vi "Autonomous Independent.vi"() -> ()   [LabVIEW 2018]
doc: "This VI is called when autonomous begins, and will automatically be terminated when autonomous ends. You can carry out timed or sensor driven robot movement independently without needing to return to the caller."
uses:
  <vilib>/Rock Robotics/WPI/RobotDrive/WPI_RobotDriveArcadeDrive_Standard(NoSaturation).vi
  <vilib>/Rock Robotics/Network Tables/NT Write Numeric Array.vi
  Robot Global Data.vi
  <vilib>/Rock Robotics/Network Tables/NT Read String.vi
panel:
  in  "Encoders":T1
  in  "PID Gains":T2={"X PID"={"proportional gain (Kc)"=0.02000000000000001, "integral time (Ti, min)"=0.0, "derivative time (Td, min)"=0.0}, "Y PID"={"proportional gain (Kc)"=0.02000000000000001, "integral time (Ti, min)"=0.0, "derivative time (Td, min)"=0.0}, "Z PID"={"proportional gain (Kc)"=0.02000000000000001, "integral time (Ti, min)"=0.0, "derivative time (Td, min)"=0.0}} {"Z PID"."derivative time (Td, min)" format="%.3f"; "Z PID"."integral time (Ti, min)" format="%.3f"; "Z PID"."proportional gain (Kc)" format="%.3f"; "Y PID"."derivative time (Td, min)" format="%.3f"; "Y PID"."integral time (Ti, min)" format="%.3f"; "Y PID"."proportional gain (Kc)" format="%.3f"; "X PID"."derivative time (Td, min)" format="%.3f"; "X PID"."integral time (Ti, min)" format="%.3f"; "X PID"."proportional gain (Kc)" format="%.3f"}
  out "Current Movement, for debugging":T3 {"Y Joystick Value" scale=1.0..-1.0; "X Joystick Value" scale=-1.0..1.0}
  in  "Array of robot movements":T4(array[cluster])=[{"X Joystick Value"=0.39393939393939403, "Y Joystick Value"=0.0, "Delay (sec)"=1.0, "Movement Name"="turn"}, {"X Joystick Value"=-0.3737373737373737, "Y Joystick Value"=0.0, "Delay (sec)"=1.0, "Movement Name"="turn back"}] {"Y Joystick Value" scale=1.0..-1.0; "X Joystick Value" scale=-1.0..1.0}
  # "Be sure to right-click and choose Data Operations>>Make Current Value default if you want to save the array values with the VI"
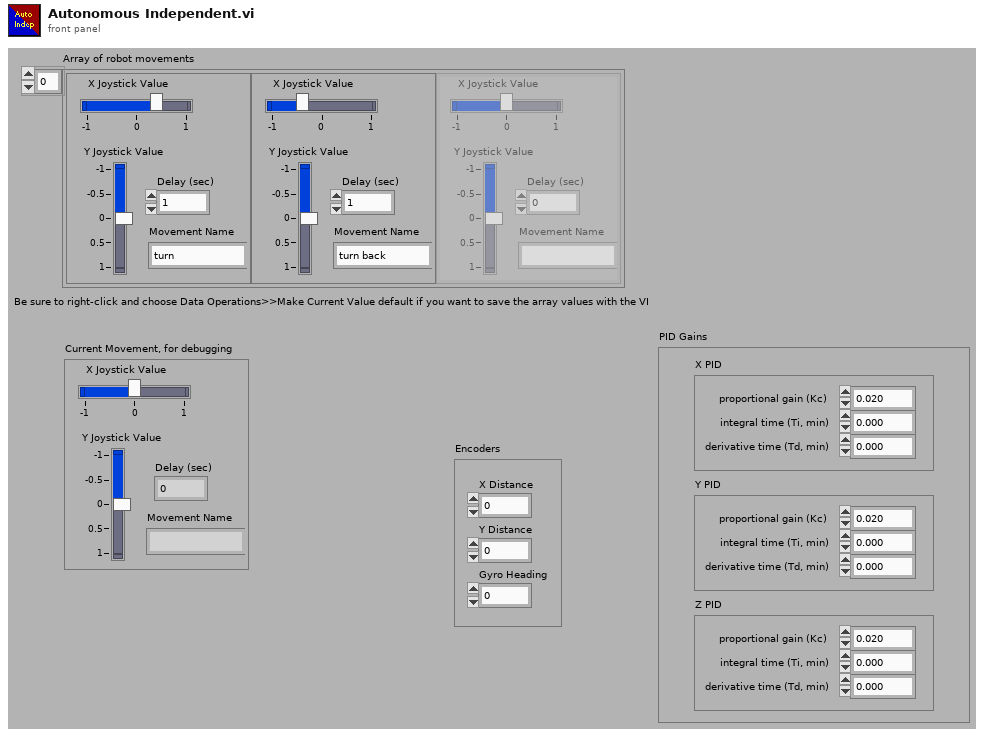
[diagram p1: front panel]
types:
  T1 = cluster{"X Distance":dbl, "Y Distance":dbl, "Gyro Heading":dbl}
  T2 = cluster{"X PID":cluster{"proportional gain (Kc)":dbl, "integral time (Ti, min)":dbl, "derivative time (Td, min)":dbl}, "Y PID":cluster{"proportional gain (Kc)":dbl, "integral time (Ti, min)":dbl, "derivative time (Td, min)":dbl}, "Z PID":cluster{"proportional gain (Kc)":dbl, "integral time (Ti, min)":dbl, "derivative time (Td, min)":dbl}}
  T3 = cluster{"X Joystick Value":dbl, "Y Joystick Value":dbl, "Delay (sec)":dbl, "Movement Name":string}
  T4 = cluster{"X Joystick Value":dbl, "Y Joystick Value":dbl, "Delay (sec)":dbl, "Movement Name":string}[]
  T5 = typedef "WPI_JoystickDevRef.ctl" = cluster{"Device":T6}
  T6 = typedef "WPI_JoystickDeviceEnum.ctl" = enum16{"USB 0", "USB 1", "USB 2", "USB 3", "USB 4", "USB 5"}
  T7 = cluster{"X Dist.":dbl, "Y Dist.":dbl, "Gyro":dbl}
  T8 = typedef "WPI_RobotDriveDevRef.ctl" = cluster{"DevStatus":errorcluster, "Motors[]":T9[], "Square Inputs":bool, "Max Output":dbl}
  T9 = typedef "WPI_MotorControlDeviceRef.ctl" = cluster{"DeviceStatus":errorcluster, "Type":T10, "PWM":cluster{"PWM Channel":T11, "DeadBand":T12}, "CAN":cluster{"Device Number":u8, "SetOutput VI Ref":variant, "GetOutput VI Ref":variant, "Enable VI Ref":variant, "Disable VI Ref":variant, "Data":variant}, "Invert":bool, "DIO PWM":cluster{"PWM \"Enable\" Channel":T11, "DIOChannel":T13, "PWM Rate":dbl}}
  T10 = typedef "WPI_MotorControlType.ctl" = enum16{"PWM", "CAN", "DIO PWM"}
  T11 = typedef "FPGA_DIOPWMChannel.ctl" = enum8{"PWM 0", "PWM 1", "PWM 2", "PWM 3", "PWM 4", "PWM 5", "PWM 6", "PWM 7", "PWM 8", "PWM 9", "PWM MXP 0", "PWM MXP 1", "PWM MXP 2", "PWM MXP 3", "PWM MXP 4", "PWM MXP 5", "PWM MXP 6", "PWM MXP 7", "PWM MXP 8", "PWM MXP 9", "Invalid"}
  T12 = typedef "WPI_PWMDeadband.ctl" = cluster{"Name":string, "maxPositivePwm":i32, "minPositivePwm":i32, "centerPwm":i32, "maxNegativePwm":i32, "minNegativePwm":i32, "angularRange":u16}
  T13 = typedef "FPGA_DIOChannel.ctl" = enum8{"DIO 0", "DIO 1", "DIO 2", "DIO 3", "DIO 4", "DIO 5", "DIO 6", "DIO 7", "DIO 8", "DIO 9", "DIO MXP 0", "DIO MXP 1", "DIO MXP 2", "DIO MXP 3", "DIO MXP 4", "DIO MXP 5", "DIO MXP 6", "DIO MXP 7", "DIO MXP 8", "DIO MXP 9", "DIO MXP 10", "DIO MXP 11", "DIO MXP 12", "DIO MXP 13", "DIO MXP 14", "DIO MXP 15", "SPI Port CS1", "SPI Port CS2", "SPI Port CS3", "SPI Port MISO", "SPI Port MOSI", "Invalid"}
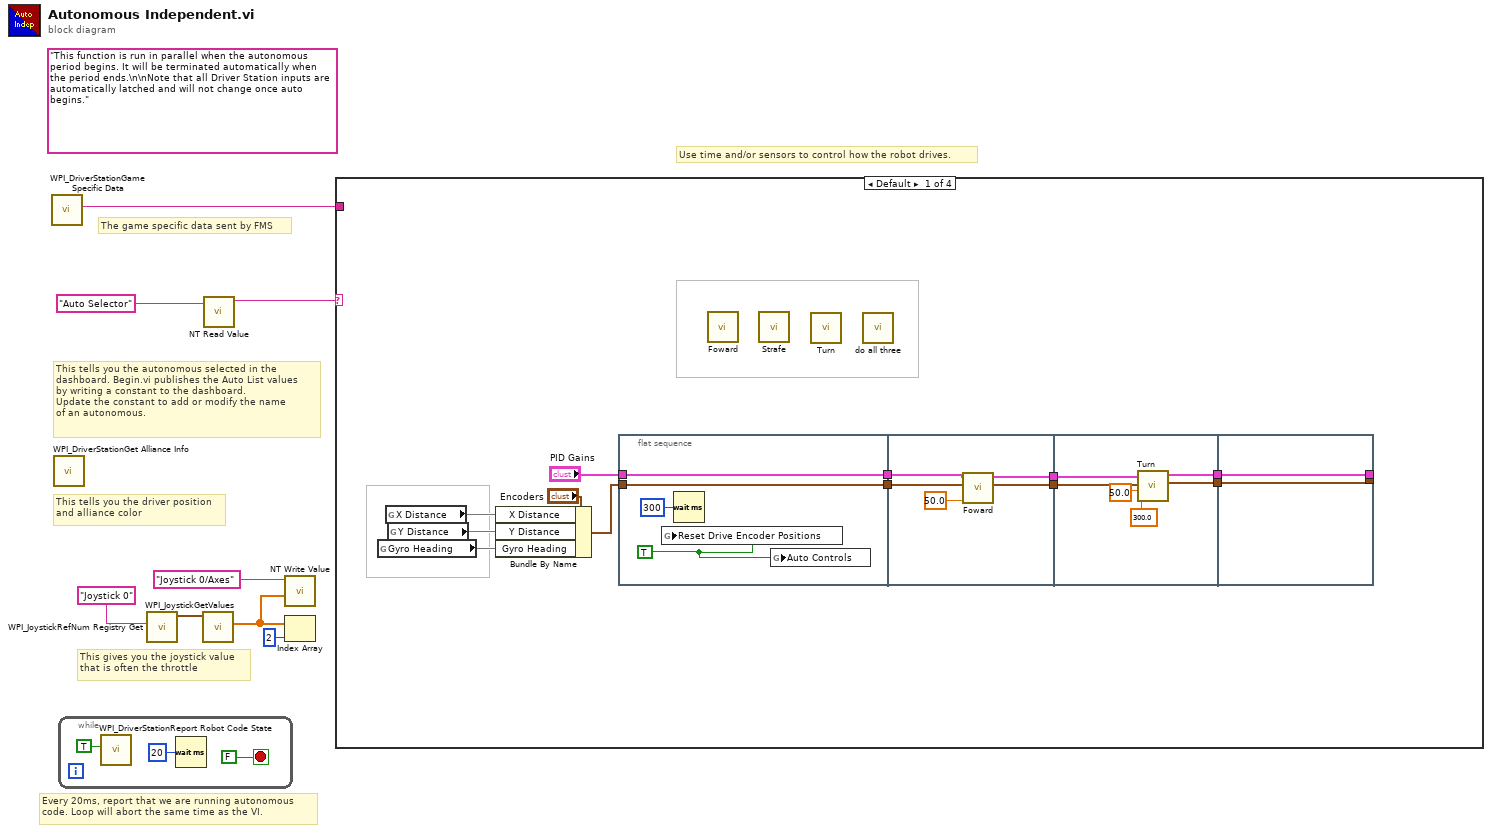
[diagram p0: block diagram]
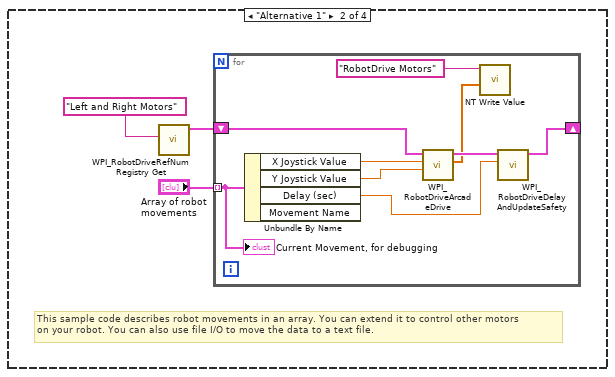
[diagram p2: hidden frame]
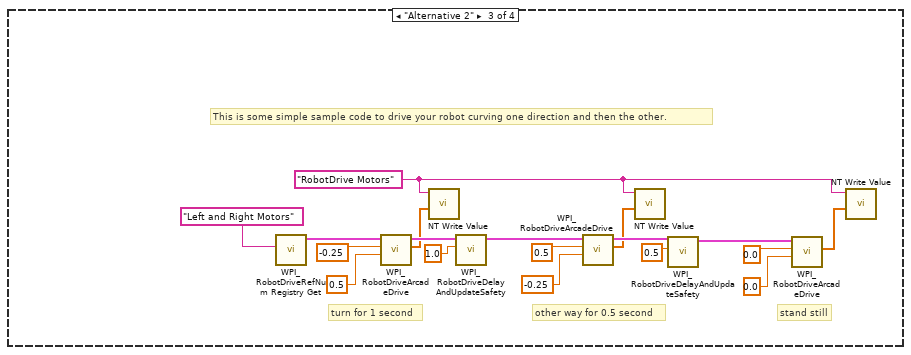
[diagram p3: hidden frame]
diagram:
  (unwired) "This function is run in parallel when the autonomous period begins. It will be terminated automatically when the period ends.\n\nNote that all Driver Station inputs are automatically latched and will not change once auto begins."
  # "The game specific data sent by FMS"
  # "This tells you the autonomous selected in the \ndashboard. Begin.vi publishes the Auto List values\nby writing a constant to the dashboard.\nUpdate the constant to add or modify the name\nof an autonomous."
  # "Every 20ms, report that we are running autonomous\ncode. Loop will abort the same time as the VI."
  # "This gives you the joystick value\nthat is often the throttle"
  # "Use time and/or sensors to control how the robot drives."
  # "This tells you the driver position\nand alliance color"
  n1 = call <vilib>:"WPI_DriverStationGame Specific Data.vi"() -> ("Game Specific Data"=w1:string)  [unwired: 11 in]
  n2 = call <vilib>:"WPI_DriverStationGet Alliance Info.vi"() -> ()  [unwired: 12 out]
  n3 = while {
    stop <- FALSE stop-if-true
    n4 = call <vilib>:"WPI_DriverStationReport Robot Code State.vi"("Autonomous"=TRUE) -> ()  [unwired: 10 in, 1 out]
    n5 = Wait (ms)(milliseconds to wait=u32 20) -> ()  [unwired: 1 out]
  }
  n6 = call <vilib>:"WPI_JoystickRefNum Registry Get.vi"("refnum name"="Joystick 0") -> ("JoystickDevRef"=w7:T5)  [unwired: 1 in, 9 out]
  n7 = call <vilib>:"WPI_JoystickGetValues.vi"("JoystickDevRef"=w7) -> ("Axes"=w3:dbl[])  [unwired: 6 in, 4 out]
  n8 = call-poly <vilib>:"NT Read Value.vi"("Name"="Auto Selector") -> ("String"=w4:string)  [unwired: 9 in, 1 out]
  n9 = call-poly <vilib>:"NT Write Value.vi"("Numeric Array"=w3, "Name"="Joystick 0/Axes") -> ()  [unwired: 9 in, 1 out]
  n10 = Index Array(array=w3, index=2) -> ()  [unwired: 1 out]
  n11 = case shown="Default" w4 {
    tunnel: w1 -> [_ _ _ _]
    frame Default {
      n12 = global read "Robot Global Data.vi" "Gyro Heading"() -> (w23)
      n13 = global read "Robot Global Data.vi" "X Distance"() -> (w21)
      n14 = global read "Robot Global Data.vi" "Y Distance"() -> (w22)
      n15 = Bundle By Name(cluster="Encoders", "X Distance"=w21, "Y Distance"=w22, "Gyro Heading"=w23) -> (w17:T1)
      n16 = flat-sequence {
        tunnel: [w25] -> w19
        tunnel: "PID Gains" -> [w25]
        tunnel: w17 -> [w24]
        tunnel: [w24] -> w16
        tunnel: w19 -> [w31]
        tunnel: w16 -> [w30]
        tunnel: [w29] -> w15
        tunnel: [w28] -> w14
        tunnel: w15 -> [w38]
        tunnel: w14 -> [w37]
        tunnel: [w36] -> w13
        tunnel: [w35] -> w12
        tunnel: [w39] -> _
        tunnel: [w40] -> _
        tunnel: w13 -> [w40]
        tunnel: w12 -> [w39]
        frame #0 {
          w27 = TRUE ("Auto Controls")
          n17 = global write "Robot Global Data.vi" "Reset Drive Encoder Positions"(w27) -> ()
          n18 = Wait (ms)(milliseconds to wait=u32 300) -> ()  [unwired: 1 out]
          n19 = global write "Robot Global Data.vi" "Auto Controls"(w27) -> ()
        }
        frame #1 {
          n20 = call "Foward.vi"("Y Target"=50.0 ("X target"), "Encoders In"=w30, "PID Gains In"=w31) -> ("Encoders Out"=w28:T7, "PID Gains Out"=w29:T2)  [unwired: 7 in]
        }
        frame #2 {
          n21 = call "Turn.vi"("Gyro Target"=300.0, "X Target"=50.0, "Encoders In"=w37, "PID Gains In"=w38) -> ("Encoders Out"=w35:T7, "PID Gains Out"=w36:T2)  [unwired: 6 in]
        }
        frame #3 {
        }
      }
      n22 = call "Foward.vi"() -> ()  [unwired: 10 in, 2 out]
      n23 = call "Strafe.vi"() -> ()  [unwired: 10 in, 2 out]
      n24 = call "Turn.vi"() -> ()  [unwired: 10 in, 2 out]
      n25 = call "do all three.vi"() -> ()  [unwired: 12 in]
    }
    frame "Alternative 1" {
      # "This sample code describes robot movements in an array. You can extend it to control other motors\non your robot. You can also use file I/O to move the data to a text file."
      n26 = call <vilib>:"WPI_RobotDriveRefNum Registry Get.vi"("refnum name"="Left and Right Motors") -> ("RobotDriveDevRef"=w42:T8)  [unwired: 1 in, 9 out]
      n27 = for {
        shift-right: [w50] -> _
        shift-left: w42 -> [w51]
        tunnel: "Array of robot movements" -> [w46] mode=indexing
        n28 = Unbundle By Name(w46) -> ("X Joystick Value"=w49:dbl, "Y Joystick Value"=w48:dbl, "Delay (sec)"=w47:dbl)  [unwired: 1 out]
        n29 = call-poly <vilib>:"WPI_RobotDriveArcadeDrive.vi"("Y axis value"=w48, "X axis value"=w49, "RobotDriveDevRef"=w51) -> ("Motor Values"=w44:dbl[], "RobotDriveDevRef"=w52:T8)  [unwired: 1 in, 6 out]
        n30 = call-poly <vilib>:"NT Write Value.vi"("Numeric Array"=w44, "Name"="RobotDrive Motors") -> ()  [unwired: 9 in, 1 out]
        n31 = call <vilib>:"WPI_RobotDriveDelayAndUpdateSafety.vi"("Delay (s)"=w47, "RobotDriveDevRef"=w52) -> ("RobotDriveDevRef 2"=w50:T8)  [unwired: 8 in, 1 out]
        "Current Movement, for debugging" <- w46
      }
    }
    frame "Alternative 2" {
      w54 = "RobotDrive Motors" ("Name")
      # "This is some simple sample code to drive your robot curving one direction and then the other."
      # "stand still"
      # "other way for 0.5 second"
      # "turn for 1 second"
      n32 = call <vilib>:"WPI_RobotDriveRefNum Registry Get.vi"("refnum name"="Left and Right Motors") -> ("RobotDriveDevRef"=w70:T8)  [unwired: 1 in, 9 out]
      n33 = call-poly <vilib>:"WPI_RobotDriveArcadeDrive.vi"("Y axis value"=0.5 ("X axis value"), "X axis value"=-0.25, "RobotDriveDevRef"=w70) -> ("Motor Values"=w53:dbl[], "RobotDriveDevRef"=w63:T8)  [unwired: 1 in, 6 out]
      n34 = call-poly <vilib>:"NT Write Value.vi"("Numeric Array"=w53, "Name"=w54) -> ()  [unwired: 9 in, 1 out]
      n35 = call <vilib>:"WPI_RobotDriveDelayAndUpdateSafety.vi"("Delay (s)"=1.0, "RobotDriveDevRef"=w63) -> ("RobotDriveDevRef 2"=w64:T8)  [unwired: 8 in, 1 out]
      n36 = call-poly <vilib>:"WPI_RobotDriveArcadeDrive.vi"("Y axis value"=-0.25 ("X axis value"), "X axis value"=0.5, "RobotDriveDevRef"=w64) -> ("Motor Values"=w55:dbl[], "RobotDriveDevRef"=w65:T8)  [unwired: 1 in, 6 out]
      n37 = call-poly <vilib>:"NT Write Value.vi"("Numeric Array"=w55, "Name"=w54) -> ()  [unwired: 9 in, 1 out]
      n38 = call <vilib>:"WPI_RobotDriveDelayAndUpdateSafety.vi"("Delay (s)"=0.5, "RobotDriveDevRef"=w65) -> ("RobotDriveDevRef 2"=w66:T8)  [unwired: 8 in, 1 out]
      n39 = call-poly <vilib>:"WPI_RobotDriveArcadeDrive.vi"("Y axis value"=0.0 ("X axis value"), "X axis value"=0.0, "RobotDriveDevRef"=w66) -> ("Motor Values"=w56:dbl[])  [unwired: 1 in, 7 out]
      n40 = call-poly <vilib>:"NT Write Value.vi"("Numeric Array"=w56, "Name"=w54) -> ()  [unwired: 9 in, 1 out]
    }
    frame "Your Turn" {
    }
  }
